vi "configuration UI.vi"() -> ()   [LabVIEW 2013, in "Modbus Slave editor node.lvclass"]
doc: "Platypus Framework 1.0.1.65\nNI Systems Engineering - National Instruments"
uses:
  Modbus Slave editor node.lvclass
  <vilib>/CEF_TreeControl/Node/NodeRef.ctl
  <vilib>/CEF_TreeControl/Node/NISE_CEF_Node.lvclass
  <vilib>/NI/AMC/Message Queue.ctl
  <vilib>/NI/AMC/Message.ctl
  <vilib>/NI/Tools/Keyed Array/KeyedArray.ctl
  <vilib>/CEF_TreeControl/Node/UserEventRef.ctl
  <vilib>/CEF_TreeControl/Controls/EventCluster.ctl
  <vilib>/NI/TBM Modules/modbus slave/configuration/Modbus Slave configuration.lvclass
  <vilib>/NI/Module Execution Interface/Engine Configuration/engine configuration.lvclass
  <vilib>/NI/Tag Bus Data Framework/Configuration Editor/Classes/Engine Parent/Engine Parent Editor Node.lvclass
  <vilib>/NI/Tag Bus/tag/tag descriptor.lvclass
  <vilib>/NI/Tag Bus/tag/Data Type.ctl
  <vilib>/NI/Tag Bus/tag/tag descriptor.lvclass/tag descriptor.ctl
  <vilib>/NI/Tag Bus Module Framework/root configuration/TBM configuration.lvclass/TBM configuration.ctl
  <vilib>/NI/TBM Modules/modbus slave/configuration/Modbus Slave configuration.lvclass/Modbus Slave configuration.ctl
  <vilib>/NI/Tag Bus/tag/write tag name.vi
  <vilib>/NI/Tag Bus/tag/write data type.vi
  <vilib>/NI/TBM Modules/modbus slave/configuration/Write port (502).vi
  <vilib>/NI/TBM Modules/modbus slave/configuration/Read modbus channels.vi
  <vilib>/NI/Tag Bus Module Framework/root configuration/Read instance name.vi
  <vilib>/NI/Tag Bus Data Framework/Configuration Editor/Classes/Module editor node/Read Module Configuration.vi
  <vilib>/NI/Tag Bus Module Framework/root configuration/create GUID.vi
  <vilib>/NI/Tag Bus Module Framework/root configuration/TBM configuration.lvclass
  <vilib>/NI/Tag Bus Module Framework/module configuration/TBM module configuration.lvclass
  <vilib>/CEF_TreeControl/NISE_CEF_TreeControl.lvlib
  <vilib>/NI/Tag Bus Data Framework/Configuration Editor/Classes/Module editor node/module editor node.lvclass
  <vilib>/NI/TBM Modules/modbus slave/module channel/Modbus Module Channel.lvclass
  <vilib>/NI/Tools/Keyed Array/Tools_KeyedArray.lvlib
  <vilib>/NI/AMC/AMC.lvlib
panel:
  in  "export":bool
  in  "Tab Control":T1(tab)
  in  "hidden_remove":bool
  in  "hidden_settings":bool
  in  "hidden_Add":bool
  in  "Remove Button":bool
  in  "Add Button":bool
  in  "channel":i32(listbox)
  in  "settings":bool
  in  "port (502)":u16=502
  in  "mapping":i32
  in  "user event":T2
  in  "main queue":T3
  in  "node ref":T4
  # "0 - Custom (User Defined)\n1 - Optimized"
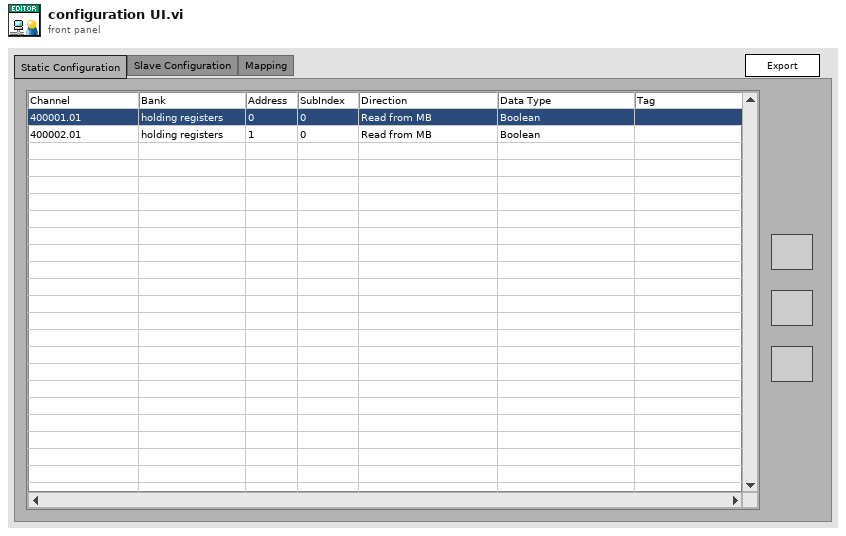
[diagram p1: front panel]
types:
  T1 = enum32{"Static Configuration", "Slave Configuration", "Mapping"}
  T2 = typedef "NISE_CEF_Node.lvclass/UserEventRef.ctl" = refnum<user-event>
  T3 = typedef "AMC.lvlib/Message Queue.ctl" = refnum<queue>
  T4 = typedef "NISE_CEF_Node.lvclass/NodeRef.ctl" = refnum<data-value>
  T5 = typedef "tag bus.lvlib/tag descriptor.lvclass/Data Type.ctl" = enum16{"Double", "Single", "I64", "I32", "I16", "I8", "U64", "U32", "U16", "U8", "Boolean", "String", "Array of Double", "Array of Single", "Array of I64", "Array of I32", "Array of I16", "Array of I8", "Array of U64", "Array of U32", "Array of U16", "Array of U8", "Array of Boolean", "Array of String"}
  T6 = typedef "NISE_CEF_TreeControl.lvlib/EventCluster.ctl" = cluster{"command":string, "data":string}
  T7 = typedef "Modbus Slave editor node.lvclass/table line.ctl" = cluster{"mbchan":refnum<class "Modbus Module Channel.lvclass">, "tag name":string}
  T8 = typedef "LVPoint32TypeDef.ctl" = cluster{"Horizontal":i32, "Vertical":i32}
  T9 = typedef "LVRowAndColumnTypeDef.ctl" = cluster{"Row":i32, "Column":i32}
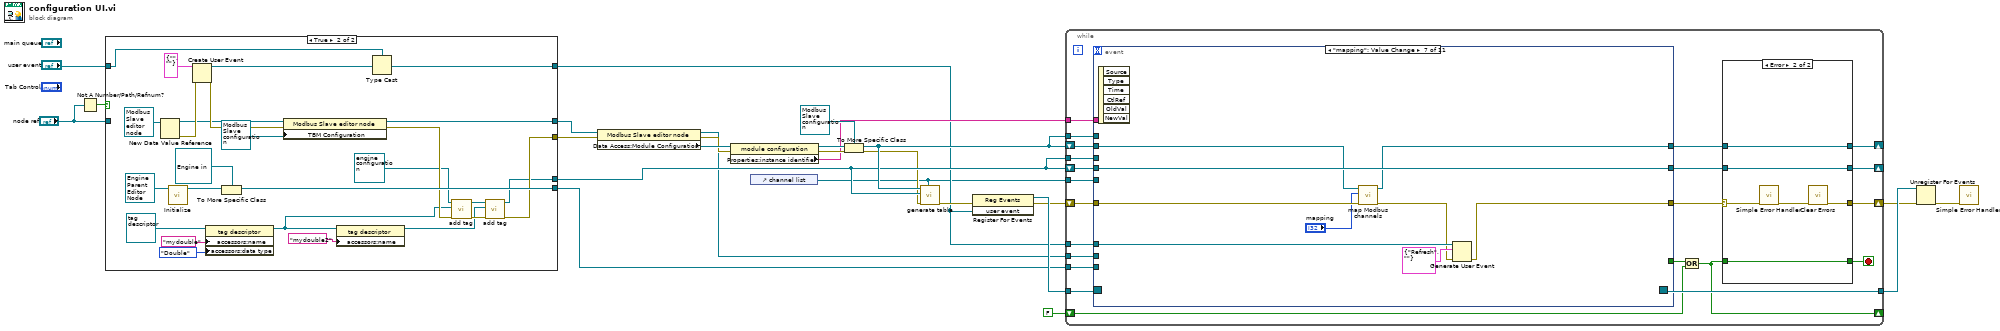
[diagram p0: block diagram]
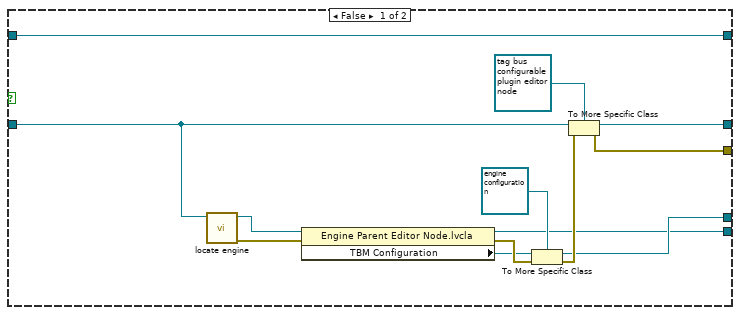
[diagram p2: hidden frame]
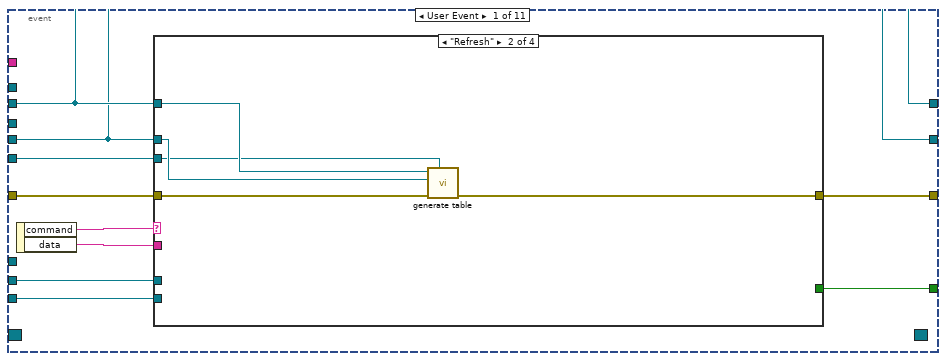
[diagram p4: hidden frame]
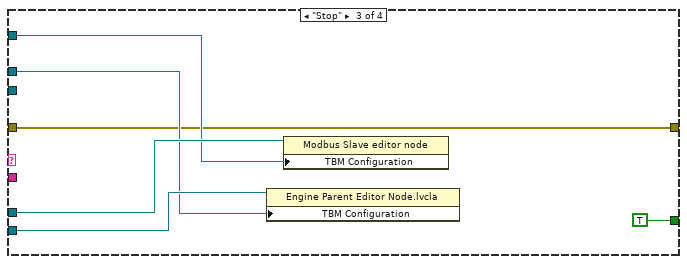
[diagram p6: hidden frame]
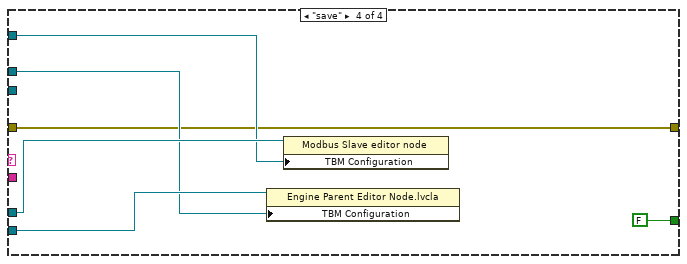
[diagram p7: hidden frame]
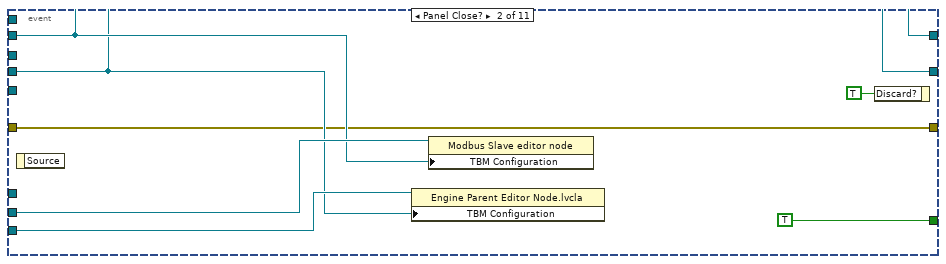
[diagram p8: hidden frame]
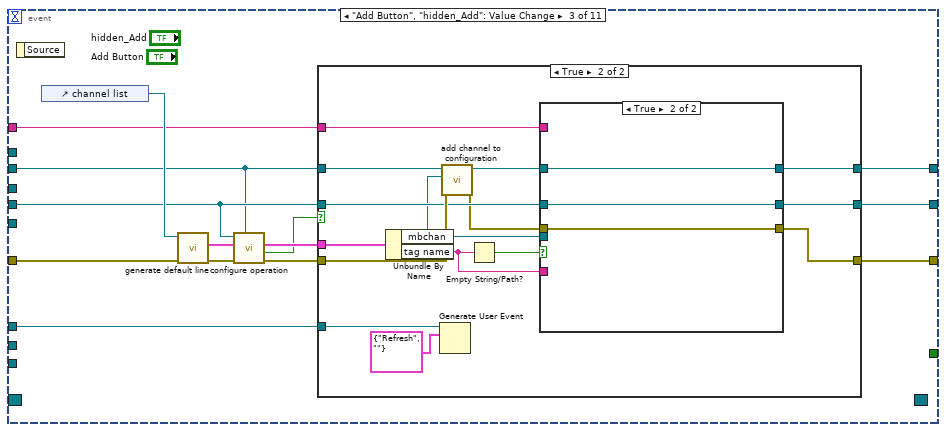
[diagram p9: hidden frame]
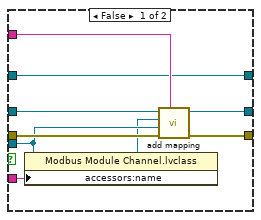
[diagram p11: hidden frame]
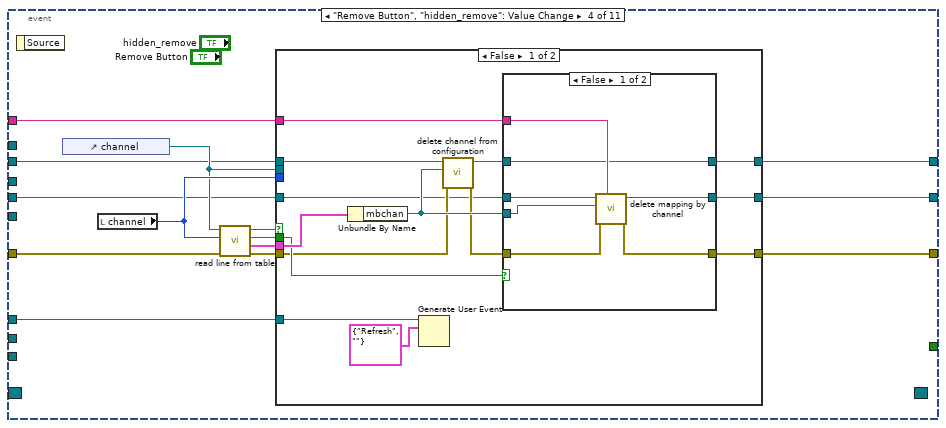
[diagram p12: hidden frame]
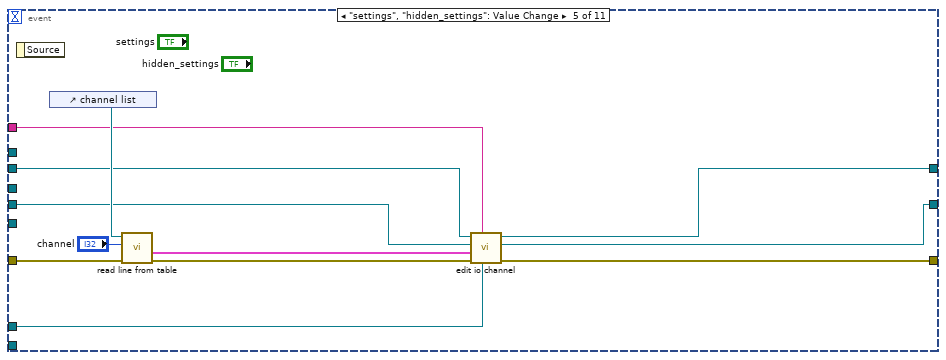
[diagram p15: hidden frame]
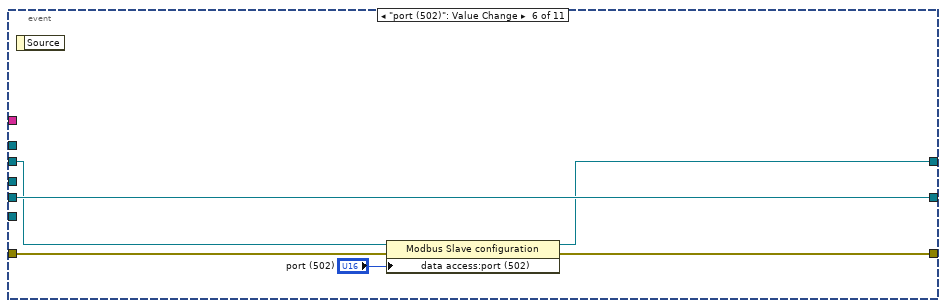
[diagram p16: hidden frame]
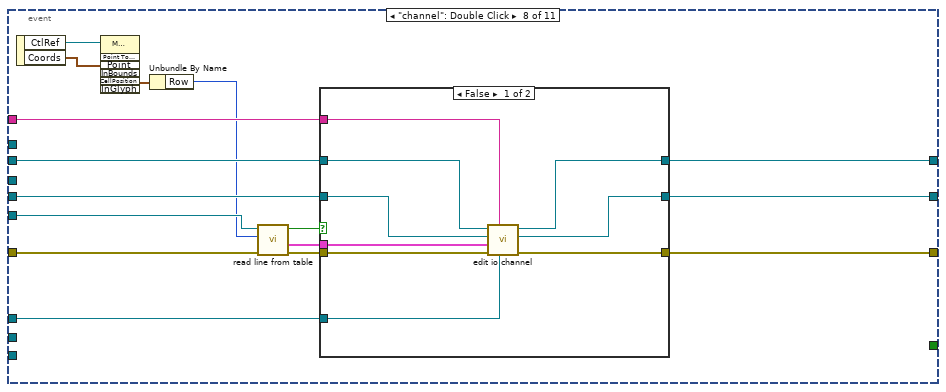
[diagram p17: hidden frame]
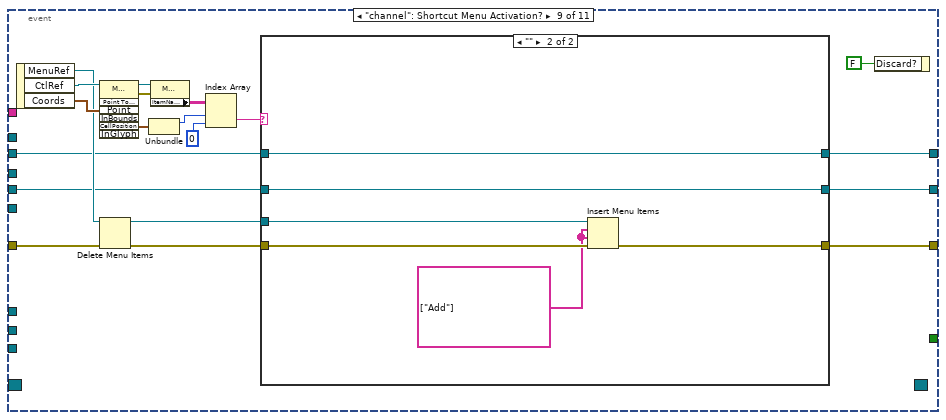
[diagram p19: hidden frame]
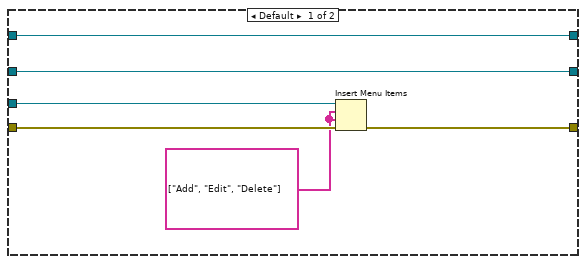
[diagram p20: hidden frame]
diagram:
  n1 = Not A Number/Path/Refnum?(number/path/refnum="node ref") -> (NaN/Path/Refnum?=w16:bool)
  n2 = case shown="True" w16 {
    tunnel: "user event" -> [w38 w40]
    tunnel: [w38 w41] -> w2
    tunnel: "node ref" -> [w36 _]
    tunnel: [w35 w58] -> w8
    tunnel: [w34 w45] -> w14
    tunnel: [w27 w44] -> w10
    tunnel: [w26 w55] -> w4
    frame False {
      n3 = call <vilib>:"locate engine.vi"("component"=w36) -> ("error out"=w31:errorcluster, "engine"=w33:refnum<data-value>)  [unwired: 9 in]
      n4 = property class="Engine Parent Editor Node.lvcla"(reference=w33, error in=w31) -> (reference out=w26:refnum<data-value>, error out=w30:errorcluster, "TBM Configuration"=w29:refnum<class "TBM configuration.lvclass">)
      n5 = To More Specific Class(target class=refnum<class "engine configuration.lvclass"> refnum ("engine configuration.lvclass"), reference=w29, error in=w30) -> (specific class reference=w27:refnum<class "engine configuration.lvclass">, error out=w28:errorcluster)
      n6 = To More Specific Class(target class=refnum<data-value> refnum ("data value reference"), reference=w36, error in=w28) -> (specific class reference=w35:refnum<data-value>, error out=w34:errorcluster)
    }
    frame True {
      n7 = New Data Value Reference(data value=refnum<class "Modbus Slave editor node.lvclass"> refnum ("tag bus configurable plugin editor node")) -> (data value reference=w57:refnum<data-value>, error out=w60:errorcluster)  [unwired: 1 in]
      n8 = call-dynamic "Initialize.vi"("Engine in"=refnum<class "Engine Parent Editor Node.lvclass"> refnum) -> ("data value reference"=w56:T4)  [unwired: 8 in, 2 out]
      n9 = Create User Event(user event datatype=T6 {"command"="", "data"=""} ("event data"), error in=w60) -> (user event=w63:refnum<user-event>, error out=w59:errorcluster)
      n10 = property class="tag descriptor"(reference=refnum<class "tag descriptor.lvclass"> refnum ("tag descriptor"), "accessors:name"="mydouble" ("name"), "accessors:data type"=Data_Type."Double" ("data type")) -> (reference out=w42:refnum<class "tag descriptor.lvclass">)  [unwired: 1 in, 1 out]
      n11 = To More Specific Class(target class=refnum<data-value> refnum ("data value reference"), reference=w56) -> (specific class reference=w55:refnum<data-value>)  [unwired: 1 in, 1 out]
      n12 = property class="Modbus Slave editor node"(reference=w57, error in=w59, "TBM Configuration"=refnum<class "Modbus Slave configuration.lvclass"> refnum ("tag bus configurable plugin module configuration")) -> (reference out=w58:refnum<data-value>, error out=w49:errorcluster)
      n13 = property class="tag descriptor"(reference=w42, "accessors:name"="mydouble2" ("name")) -> (reference out=w43:refnum<class "tag descriptor.lvclass">)  [unwired: 1 in, 1 out]
      n14 = Type Cast(type=w40, x=w63) -> (*(type *) &x=w41:T2)
      n15 = call <vilib>:"add tag.vi"("error in"=w49, "tag descriptor"=w42, "engine configuration in"=refnum<class "engine configuration.lvclass"> refnum ("Engine Configuration")) -> ("error out"=w47:errorcluster, "engine configuration out"=w46:refnum<class "engine configuration.lvclass">)  [unwired: 7 in]
      n16 = call <vilib>:"add tag.vi"("error in"=w47, "tag descriptor"=w43, "engine configuration in"=w46) -> ("error out"=w45:errorcluster, "engine configuration out"=w44:refnum<class "engine configuration.lvclass">)  [unwired: 7 in]
    }
  }
  n17 = property class="Modbus Slave editor node"(reference=w8, error in=w14) -> (reference out=w5:refnum<data-value>, error out=w19:errorcluster, "Data Access:Module Configuration"=w20:refnum<class "TBM module configuration.lvclass">)
  n18 = property class="module configuration"(reference=w20, error in=w19) -> (reference out=w17:refnum<class "TBM module configuration.lvclass">, error out=w18:errorcluster, "Properties:instance identifier"=w13:string)
  n19 = control-ref of="channel list"() -> (w1:refnum<vi>)
  n20 = To More Specific Class(target class=refnum<class "Modbus Slave configuration.lvclass"> refnum ("tag bus configurable plugin module configuration"), reference=w17, error in=w18) -> (specific class reference=w11:refnum<class "Modbus Slave configuration.lvclass">, error out=w9:errorcluster)
  n21 = call "generate table.vi"("table"=w1, "error in"=w9, "engine configuration"=w10, "tag bus configurable plugin module configuration"=w11) -> ("error out"=w7:errorcluster)  [unwired: 7 in]
  n22 = register-events(error in=w7, w2) -> (reference out=w25:refnum<event-registration>, error out=w6:errorcluster)  [unwired: 1 in]
  n23 = while {
    tunnel: w25 -> [w86]
    tunnel: [w85] -> w24
    shift-right: [w79] -> w23
    shift-left: w6 -> [w84]
    shift-right: [w81] -> _
    shift-left: FALSE -> [w80]
    tunnel: w11 -> [w77]
    shift-right: [w73] -> _
    shift-left: w11 -> [w78]
    shift-right: [w74] -> _
    shift-left: w10 -> [w75]
    tunnel: w10 -> [w76]
    tunnel: w13 -> [w72]
    tunnel: w5 -> [w69]
    tunnel: w4 -> [w68]
    tunnel: w2 -> [w67]
    tunnel: w1 -> [w65]
    stop <- w83 stop-if-true
    n24 = event shown="[6] \"mapping\": Value Change" {
      selector: w86 -> [_ _ _ _ _ _ _ _ _ _ _]
      dyn-events: [_ _ _ _ _ _ _ _ _ _ _] -> w85
      timeout: _ -> [_ _ _ _ _ _ _ _ _ _ _]
      tunnel: [w106 TRUE _ _ _ _ _ _ _ _ _] -> w82
      tunnel: [w98 w126 w145 w189 w227 w232 w235 w258 w272 w307 w335] -> w66
      tunnel: w84 -> [w99 w126 w144 w188 w228 w234 w243 w259 w290 w306 w340]
      tunnel: w78 -> [w102 w128 w132 w184 w221 w231 w241 w254 w279 w311 w341]
      tunnel: w77 -> [_ _ _ _ _ _ _ _ _ _ _]
      tunnel: w76 -> [_ _ _ _ _ _ _ _ _ _ _]
      tunnel: w75 -> [w101 w127 w133 w183 w222 w233 w242 w255 w275 w310 w342]
      tunnel: [w101 w127 w138 w178 w219 w233 w242 w252 w276 w308 w342] -> w71
      tunnel: [w102 w128 w137 w177 w220 w230 w240 w253 w277 w309 w334] -> w70
      tunnel: w72 -> [_ _ w136 w179 w218 _ _ w251 _ _ _]
      tunnel: w69 -> [w104 w130 _ _ _ _ _ _ _ _ _]
      tunnel: w68 -> [w103 w129 _ _ _ _ _ _ _ _ _]
      tunnel: w67 -> [_ _ w134 w176 w217 _ w237 w250 _ _ _]
      tunnel: w65 -> [w97 _ _ _ _ _ _ w249 _ _ _]
      event User Event {
        n25 = event-data() -> ("command"=w105:string, "data"=w100:string)  [unwired: 1 in]
        n26 = case shown="\"Refresh\"" w105 {
          tunnel: [_ _ TRUE FALSE] -> w106
          tunnel: w104 -> [_ _ w117 w123]
          tunnel: w103 -> [_ _ w116 w122]
          tunnel: w102 -> [_ w112 w115 w121]
          tunnel: w101 -> [_ w111 w114 w120]
          tunnel: w100 -> [_ _ _ _]
          tunnel: w99 -> [w107 w110 w113 w119]
          tunnel: [w107 w109 w113 w119] -> w98
          tunnel: w97 -> [_ w108 _ _]
          frame Default {
          }
          frame "Refresh" {
            n27 = call "generate table.vi"("table"=w108, "error in"=w110, "engine configuration"=w111, "tag bus configurable plugin module configuration"=w112) -> ("error out"=w109:errorcluster)  [unwired: 7 in]
          }
          frame "Stop" {
            n28 = property class="Engine Parent Editor Node.lvcla"(reference=w116, "TBM Configuration"=w114) -> ()  [unwired: 1 in, 2 out]
            n29 = property class="Modbus Slave editor node"(reference=w117, "TBM Configuration"=w115) -> ()  [unwired: 1 in, 2 out]
          }
          frame "save" {
            n30 = property class="Engine Parent Editor Node.lvcla"(reference=w122, "TBM Configuration"=w120) -> ()  [unwired: 1 in, 2 out]
            n31 = property class="Modbus Slave editor node"(reference=w123, "TBM Configuration"=w121) -> ()  [unwired: 1 in, 2 out]
          }
        }
      }
      event Panel Close? {
        n32 = event-data() -> ()  [unwired: 1 in, 1 out]
        n33 = property class="Engine Parent Editor Node.lvcla"(reference=w129, "TBM Configuration"=w127) -> ()  [unwired: 1 in, 2 out]
        n34 = property class="Modbus Slave editor node"(reference=w130, "TBM Configuration"=w128) -> ()  [unwired: 1 in, 2 out]
        n35 = event-data("Discard?"=TRUE) -> ()  [unwired: 1 in, 1 out]
      }
      event "Add Button", "hidden_Add": Value Change {
        n36 = event-data() -> ()  [unwired: 1 in, 1 out]
        n37 = control-ref of="channel list"() -> (w143:refnum<vi>)
        n38 = call "generate default line.vi"("error in"=w144, "operations table"=w143) -> ("error out"=w141:errorcluster, "line"=w142:T7)  [unwired: 8 in]
        n39 = call "configure operation.vi"("tag bus configurable plugin module configuration"=w132, "error in"=w141, "line item in"=w142, "engine configuration"=w133) -> ("error out"=w139:errorcluster, "success"=w135:bool, "line item out"=w140:T7)  [unwired: 4 in, 1 out]
        n40 = case shown="True" w135 {
          tunnel: [w148 w151] -> w145
          tunnel: w139 -> [w148 w161]
          tunnel: w133 -> [w147 w159]
          tunnel: w140 -> [_ w162]
          tunnel: w132 -> [w146 w163]
          tunnel: [w147 w158] -> w138
          tunnel: [w146 w152] -> w137
          tunnel: w136 -> [_ w155]
          tunnel: w134 -> [_ w150]
          frame False {
          }
          frame True {
            n41 = Unbundle By Name(w162) -> ("mbchan"=w156:refnum<class "Modbus Module Channel.lvclass">, "tag name"=w154:string)
            n42 = Generate User Event(user event=w150, event data cluster=T6 {"command"="Refresh", "data"=""} ("event data")) -> ()  [unwired: 2 in, 2 out]
            n43 = call <vilib>:"add channel to configuration.vi"("error in"=w161, "Modbus Module Channel.lvclass"=w156, "Modbus Slave configuration in"=w163) -> ("error out"=w157:errorcluster, "Modbus Slave configuration out"=w153:refnum<class "Modbus Slave configuration.lvclass">)  [unwired: 7 in]
            n44 = Empty String/Path?(string/path=w154) -> (empty?=w160:bool)
            n45 = case shown="True" w160 {
              tunnel: w159 -> [w172 w175]
              tunnel: [w171 w175] -> w158
              tunnel: w157 -> [w170 w174]
              tunnel: w156 -> [w168 _]
              tunnel: w155 -> [w169 _]
              tunnel: w154 -> [w167 _]
              tunnel: [w165 w174] -> w151
              tunnel: w153 -> [w164 w173]
              tunnel: [w164 w173] -> w152
              frame False {
                n46 = property class="Modbus Module Channel.lvclass"(reference=w168, "accessors:name"=w167) -> (reference out=w166:refnum<class "Modbus Module Channel.lvclass">)  [unwired: 1 in, 1 out]
                n47 = call <vilib>:"add mapping.vi"("owner ID"=w169, "error in"=w170, "channel"=w168, "tag descriptor"=w166, "engine configuration"=w172) -> ("error out"=w165:errorcluster, "engine configuration out"=w171:refnum<class "engine configuration.lvclass">)  [unwired: 5 in]
              }
              frame True {
              }
            }
          }
        }
      }
      event "Remove Button", "hidden_remove": Value Change {
        n48 = event-data() -> ()  [unwired: 1 in, 1 out]
        n49 = control-ref of="channel"() -> (w186:refnum<vi>)
        n50 = local read "channel"() -> (w187:i32)
        n51 = call "read line from table.vi"("error in"=w188, "line number"=w187, "channels table"=w186) -> ("error out"=w180:errorcluster, "line"=w185:T7, "empty tag?"=w181:bool, "empty channel?"=w182:bool)  [unwired: 5 in]
        n52 = case shown="False" w182 {
          tunnel: [w192 w215] -> w189
          tunnel: w187 -> [_ _]
          tunnel: w186 -> [_ _]
          tunnel: w185 -> [w203 _]
          tunnel: w184 -> [w201 w214]
          tunnel: w183 -> [w196 w216]
          tunnel: w181 -> [w202 _]
          tunnel: w180 -> [w199 w215]
          tunnel: w179 -> [w195 _]
          tunnel: [w194 w216] -> w178
          tunnel: [w193 w214] -> w177
          tunnel: w176 -> [w190 _]
          frame False {
            n53 = Unbundle By Name(w203) -> ("mbchan"=w200:refnum<class "Modbus Module Channel.lvclass">)
            n54 = Generate User Event(user event=w190, event data cluster=T6 {"command"="Refresh", "data"=""} ("event data")) -> ()  [unwired: 2 in, 2 out]
            n55 = call <vilib>:"delete channel from configuration.vi"("error in"=w199, "Modbus Module Channel.lvclass"=w200, "Modbus Slave configuration in"=w201) -> ("error out"=w197:errorcluster, "Modbus Slave configuration out"=w198:refnum<class "Modbus Slave configuration.lvclass">)  [unwired: 7 in]
            n56 = case shown="False" w202 {
              tunnel: w200 -> [w209 _]
              tunnel: w198 -> [w204 w211]
              tunnel: w197 -> [w207 w212]
              tunnel: w196 -> [w210 w213]
              tunnel: w195 -> [w208 _]
              tunnel: [w206 w213] -> w194
              tunnel: [w205 w212] -> w192
              tunnel: [w204 w211] -> w193
              frame False {
                n57 = call <vilib>:"delete mapping by channel.vi"("owner ID"=w208, "error in"=w207, "channel"=w209, "engine configuration in"=w210) -> ("error out"=w205:errorcluster, "engine configuration out"=w206:refnum<class "engine configuration.lvclass">)  [unwired: 6 in]
              }
              frame True {
              }
            }
          }
          frame True {
          }
        }
      }
      event "settings", "hidden_settings": Value Change {
        n58 = event-data() -> ()  [unwired: 1 in, 1 out]
        n59 = control-ref of="channel list"() -> (w226:refnum<vi>)
        n60 = call "read line from table.vi"("error in"=w228, "line number"="channel", "channels table"=w226) -> ("error out"=w225:errorcluster, "line"=w224:T7)  [unwired: 5 in, 2 out]
        n61 = call "edit io channel.vi"("user event"=w217, "Properties:instance identifier"=w218, "error in"=w225, "line"=w224, "engine configuration in"=w222, "tag bus configurable plugin module configuration in"=w221) -> ("error out"=w227:errorcluster, "engine configuration"=w219:refnum<class "engine configuration.lvclass">, "tag bus configurable plugin module configuration out"=w220:refnum<class "Modbus Slave configuration.lvclass">)  [unwired: 3 in]
      }
      event "port (502)": Value Change {
        n62 = event-data() -> ()  [unwired: 1 in, 1 out]
        n63 = property class="Modbus Slave configuration"(reference=w231, error in=w234, "data access:port (502)"="port (502)") -> (reference out=w230:refnum<class "Modbus Slave configuration.lvclass">, error out=w232:errorcluster)
      }
      event "mapping": Value Change {
        n64 = event-data() -> ()  [unwired: 1 in, 6 out]
        n65 = call <vilib>:"map Modbus channels.vi"("error in (no error)"=w243, "mapping"="mapping", "Modbus Slave configuration in"=w241) -> ("error out"=w236:errorcluster, "Modbus Slave configuration out"=w240:refnum<class "Modbus Slave configuration.lvclass">)  [unwired: 7 in]
        n66 = Generate User Event(user event=w237, event data cluster=T6 {"command"="Refresh", "data"=""} ("event data"), error in=w236) -> (error out=w235:errorcluster)  [unwired: 1 in, 1 out]
      }
      event "channel": Double Click {
        n67 = event-data() -> ("CtlRef"=w248:refnum<vi>, "Coords"=w247:T8)  [unwired: 1 in]
        n68 = invoke class="MCListbox (strict)" method="Point To Row Column"(reference=w248, "Point"=w247) -> ("CellPosition"=w246:T9)  [unwired: 5 in, 6 out]
        n69 = Unbundle By Name(w246) -> ("Row"=w245:i32)
        n70 = call "read line from table.vi"("error in"=w259, "line number"=w245, "channels table"=w249) -> ("error out"=w257:errorcluster, "line"=w256:T7, "empty channel?"=w244:bool)  [unwired: 5 in, 1 out]
        n71 = case shown="False" w244 {
          tunnel: [w268 w269] -> w258
          tunnel: w257 -> [w267 w269]
          tunnel: w256 -> [w266 _]
          tunnel: w255 -> [w265 w270]
          tunnel: w254 -> [w264 w271]
          tunnel: [w263 w271] -> w253
          tunnel: [w262 w270] -> w252
          tunnel: w251 -> [w261 _]
          tunnel: w250 -> [w260 _]
          frame False {
            n72 = call "edit io channel.vi"("user event"=w260, "Properties:instance identifier"=w261, "error in"=w267, "line"=w266, "engine configuration in"=w265, "tag bus configurable plugin module configuration in"=w264) -> ("error out"=w268:errorcluster, "engine configuration"=w262:refnum<class "engine configuration.lvclass">, "tag bus configurable plugin module configuration out"=w263:refnum<class "Modbus Slave configuration.lvclass">)  [unwired: 3 in]
          }
          frame True {
          }
        }
      }
      event "channel": Shortcut Menu Activation? {
        n73 = event-data() -> ("MenuRef"=w286:refnum<k9>, "CtlRef"=w288:refnum<vi>, "Coords"=w287:T8)  [unwired: 1 in]
        n74 = invoke class="MCListbox (strict)" method="Point To Row Column"(reference=w288, "Point"=w287) -> (reference out=w285:refnum<vi>, error out=w284:errorcluster, "CellPosition"=w283:T9)  [unwired: 5 in, 4 out]
        n75 = Delete Menu Items(6:w290, 9:w286) -> (0:w273:errorcluster, 3:w274:refnum<k9>)  [unwired: 2 in]
        n76 = Unbundle(w283) -> ("Row"=w281:i32)  [unwired: 1 out]
        n77 = property class="MCListbox (strict)"(reference=w285, error in=w284) -> ("ItemNames"=w282:string[][])  [unwired: 2 out]
        n78 = Index Array(array=w282, index (row)=w281, index (col)=0 ("disabled index (col)")) -> (element=w278:string)
        n79 = case shown="\"\"" w278 {
          tunnel: w279 -> [w296 w302]
          tunnel: [w296 w302] -> w277
          tunnel: [w295 w301] -> w276
          tunnel: w275 -> [w295 w301]
          tunnel: w274 -> [w294 w300]
          tunnel: w273 -> [w293 w299]
          tunnel: [w292 w298] -> w272
          frame Default {
            w291 = string[] ["Add", "Edit", "Delete"] ("item names")
            n80 = Insert Menu Items(6:w293, 7:w291, 8:w291, 9:w294) -> (0:w292:errorcluster)  [unwired: 2 in, 2 out]
          }
          frame "" {
            w297 = string[] ["Add"] ("item names")
            n81 = Insert Menu Items(6:w299, 7:w297, 8:w297, 9:w300) -> (0:w298:errorcluster)  [unwired: 2 in, 2 out]
          }
        }
        n82 = event-data("Discard?"=FALSE) -> ()  [unwired: 1 in, 1 out]
      }
      event "channel": Shortcut Menu Selection (User) {
        n83 = event-data() -> ("ItemTag"=w312:string, "CtlRef"=w313:refnum<vi>, "Coords"=w314:T8)  [unwired: 1 in]
        n84 = invoke class="MCListbox (strict)" method="Point To Row Column"(reference=w313, "Point"=w314) -> ("CellPosition"=w304:T9)  [unwired: 5 in, 6 out]
        n85 = Unbundle By Name(w304) -> ("Row"=w303:i32)
        n86 = property on="channel" class="MCListbox (strict)"(error in=w306, "Value"=w303) -> (error out=w305:errorcluster)  [unwired: 1 in, 1 out]
        n87 = case shown="\"Delete\"" w312 {
          tunnel: w305 -> [w315 w319 w325 w330]
          tunnel: w311 -> [w317 w322 w327 w332]
          tunnel: w310 -> [w316 w321 w326 w331]
          tunnel: [w317 w322 w327 w332] -> w309
          tunnel: [w316 w321 w326 w331] -> w308
          tunnel: [w315 w318 w324 w329] -> w307
          frame Default {
          }
          frame "Add" {
            n88 = property on="hidden_Add" class="Bool (strict)"(error in=w319, "Val(Sgnl)"=TRUE ("Value (Signaling)")) -> (error out=w318:errorcluster)  [unwired: 1 in, 1 out]
          }
          frame "Edit" {
            n89 = property on="hidden_settings" class="Bool (strict)"(error in=w325, "Val(Sgnl)"=TRUE ("Value (Signaling)")) -> (error out=w324:errorcluster)  [unwired: 1 in, 1 out]
          }
          frame "Delete" {
            n90 = property on="hidden_remove" class="Bool (strict)"(error in=w330, "Val(Sgnl)"=FALSE ("Value (Signaling)")) -> (error out=w329:errorcluster)  [unwired: 1 in, 1 out]
          }
        }
      }
      event "export": Value Change {
        n91 = event-data() -> ()  [unwired: 1 in, 1 out]
        n92 = property class="Modbus Slave configuration"(reference=w341) -> (reference out=w334:refnum<class "Modbus Slave configuration.lvclass">, "data access:modbus channels"=w333:refnum<class "Modbus Module Channel.lvclass">[])  [unwired: 1 in, 1 out]
        n93 = call "File Dialog"("error in"=w340, "pattern (all files)"="*.csv") -> ("selected path"=w339:path, "cancelled"=w336:bool, "error out"=w337:errorcluster)  [unwired: 10 in, 1 out]
        n94 = case shown="False" w336 {
          tunnel: w339 -> [w343 _]
          tunnel: w337 -> [w345 w347]
          tunnel: [w346 w347] -> w335
          tunnel: w333 -> [w344 _]
          frame False {
            n95 = call "export csv to kepserverex.vi"("error in"=w345, "modbus channels"=w344, "selected path"=w343) -> ("error out"=w346:errorcluster)  [unwired: 8 in]
          }
          frame True {
          }
        }
      }
    }
    n96 = Or(x=w82, y=w80) -> (x .or. y?=w81:bool)
    n97 = case shown="Error" w66 {
      selector: w66 -> [w87 w95]
      tunnel: [w90 w96] -> w83
      tunnel: w81 -> [w90 w96]
      tunnel: [w87 w93] -> w79
      tunnel: w71 -> [w88 w92]
      tunnel: [w88 w92] -> w74
      tunnel: w70 -> [w89 w91]
      tunnel: [w89 w91] -> w73
      frame No Error {
      }
      frame Error {
        n98 = call <vilib>:"Simple Error Handler.vi"("error in (no error)"=w95) -> ("error out"=w94:errorcluster)  [unwired: 4 in, 4 out]
        n99 = call <vilib>:"Clear Errors.vi"("error in (no error)"=w94) -> ("error out"=w93:errorcluster)  [unwired: 6 in]
      }
    }
  }
  n100 = Unregister For Events(event registration refnum=w24, error in=w23) -> (error out=w3:errorcluster)
  n101 = call <vilib>:"Simple Error Handler.vi"("error in (no error)"=w3) -> ()  [unwired: 4 in, 5 out]
